vi "Stop.vi"(8 "error in (no error)":errorcluster, 11 "Application Command in":refnum<class "Application Command.lvclass">) -> (0 "error out":errorcluster, 2 "Stop":bool, 3 "Application Command out":refnum<class "Application Command.lvclass">)   [LabVIEW 2020, in "Application Command.lvclass"]
uses:
  Application Command.lvclass
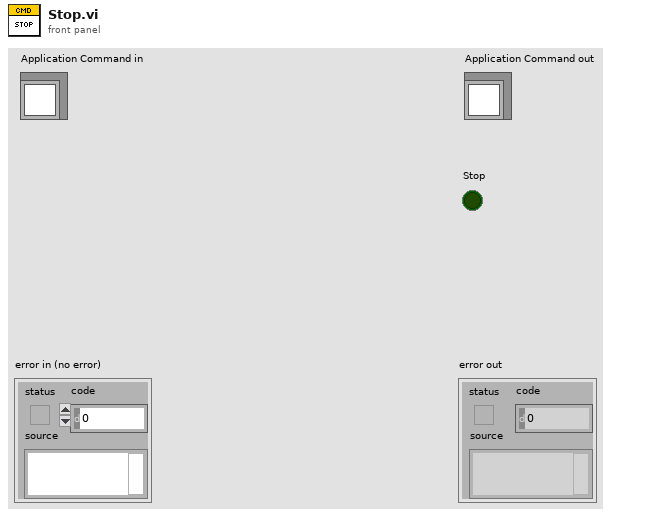
[diagram p1: front panel]
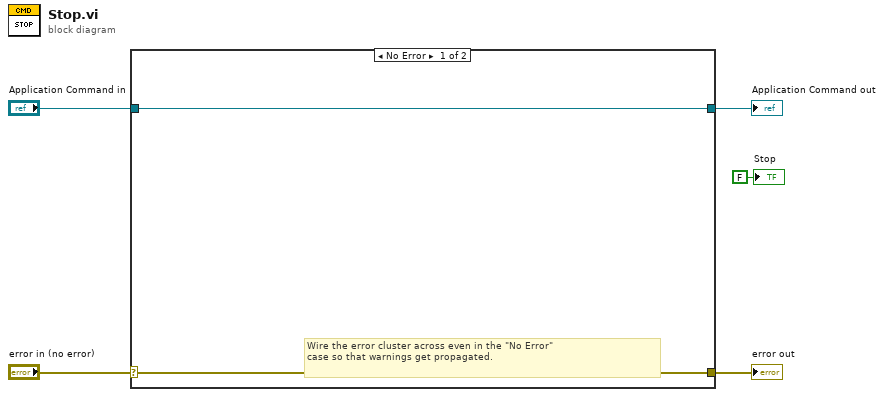
[diagram p0: block diagram]
diagram:
  n1 = case shown="No Error" "error in (no error)" {
    selector: "error in (no error)" -> [w6 w9]
    tunnel: [w6 w9] -> w4
    tunnel: [w7 w8] -> w2
    tunnel: "Application Command in" -> [w7 w8]
    frame No Error {
      # "Wire the error cluster across even in the \"No Error\"\ncase so that warnings get propagated."
    }
    frame Error {
    }
  }
  "error out" <- w4
  "Application Command out" <- w2
  "Stop" <- FALSE ("Stop")
